vi "DrawCursorLines(SubVI).vi"(11 "CtlRef":refnum<vi>) -> (2 "Array":dbl[][](array[numeric]), 3 "reference out":refnum<vi>)   [LabVIEW 2013, in "main.lvlib"]
uses:
  main.lvlib
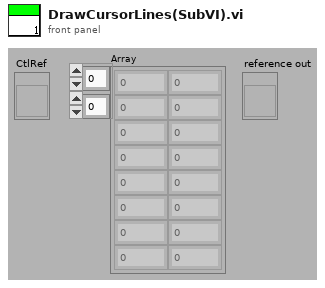
[diagram p1: front panel]
types:
  T1 = cluster{"Width":u16, "Style":enum32{"Solid", "Dash", "Dot", "DashDot", "DashDotDot"}}
  T2 = typedef "LVCursorListTypeDef.ctl" = cluster{"Name":string, "Color":u32, "Style":u8, "Point Style":u8, "Name Visible":bool, "Allow Drag":bool, "Cursor Mode":u32, "Plot":i32, "Index":i32, "Position":cluster{"X":dbl, "Y":dbl}, "X Scale":u32, "Y Scale":u32, "Watch Plots":i32[], "Watch All Plots":bool, "Plot Area":i32, "Label Offset":cluster{"X":dbl, "Y":dbl}}[]
  T3 = typedef "LVRectTypeDef.ctl" = cluster{"Left":i16, "Top":i16, "Right":i16, "Bottom":i16}
  T4 = typedef "LVPoint32TypeDef.ctl" = cluster{"Horizontal":i32, "Vertical":i32}
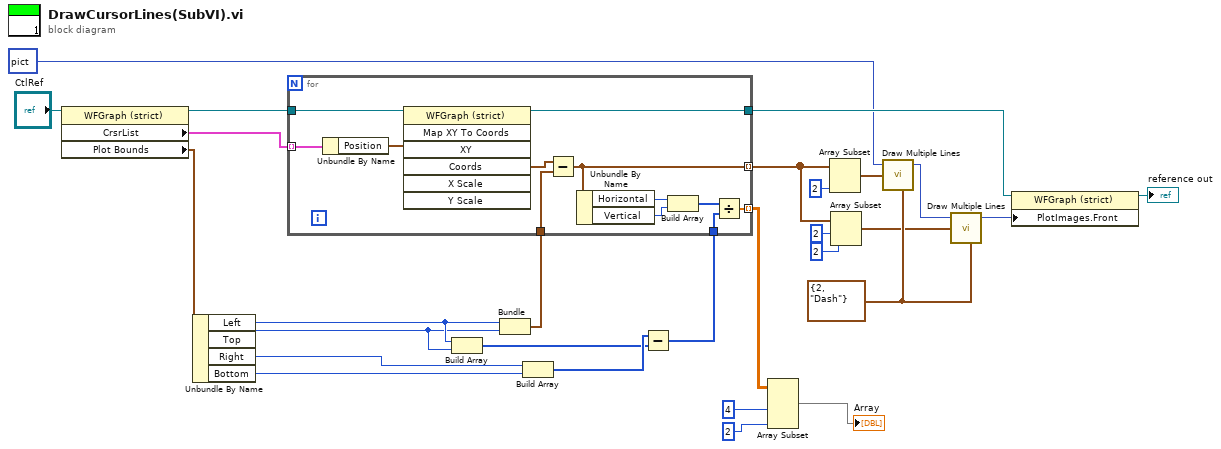
[diagram p0: block diagram]
diagram:
  w28 = T1 {"Width"=2, "Style"=enum."Dash"} ("pen")
  n1 = property class="WFGraph (strict)"(reference="CtlRef") -> (reference out=w18:refnum<vi>, "CrsrList"=w21:T2, "Plot Bounds"=w14:T3)  [unwired: 1 in, 1 out]
  n2 = Unbundle By Name(w14) -> ("Left"=w5:i16, "Top"=w4:i16, "Right"=w7:i16, "Bottom"=w8:i16)
  n3 = Build Array(w5, w4) -> (w1:i16[])
  n4 = Bundle("Left"=w5, "Top"=w4) -> (w13:cluster{"Left":i16, "Top":i16})  [unwired: 1 in]
  n5 = Build Array(w7, w8) -> (w2:i16[])
  n6 = Subtract(x=w2, y=w1) -> (x-y=w3:i16[])
  n7 = for {
    tunnel: w18 -> [w40]
    tunnel: w21 -> [w39] mode=indexing
    tunnel: w13 -> [w35]
    tunnel: [w34] -> w15 mode=indexing
    tunnel: [w37] -> w20
    tunnel: [w31] -> w6 mode=indexing
    tunnel: w3 -> [w29]
    n8 = Unbundle By Name(w39) -> ("Position"=w38:cluster{"X":dbl, "Y":dbl})
    n9 = invoke class="WFGraph (strict)" method="Map XY To Coords"(reference=w40, "XY"=w38) -> (reference out=w37:refnum<vi>, "Coords"=w36:T4)  [unwired: 5 in, 5 out]
    n10 = Subtract(x=w36, y=w35) -> (x-y=w34:T4)
    n11 = Unbundle By Name(w34) -> ("Horizontal"=w33:i32, "Vertical"=w32:i32)
    n12 = Build Array(w33, w32) -> (w30:i32[])
    n13 = Divide(x=w30, y=w29) -> (x/y=w31:dbl[])
  }
  n14 = Array Subset(array=w6, length (row)=4, length (col)=2) -> (→"Array":dbl[][])  [unwired: 2 in]
  n15 = Array Subset(array=w15, length=2) -> (w23:T4[])  [unwired: 1 in]
  n16 = Array Subset(array=w15, index=2, length=2) -> (w16:T4[])
  n17 = call <vilib>:"Draw Multiple Lines.vi"("picture"=picture data[5B] ("empty picture"), "line endpoints"=w23, "pen"=w28) -> ("new picture"=w26:picture)  [unwired: 6 in]
  n18 = call <vilib>:"Draw Multiple Lines.vi"("picture"=w26, "line endpoints"=w16, "pen"=w28) -> ("new picture"=w27:picture)  [unwired: 6 in]
  n19 = property class="WFGraph (strict)"(reference=w20, "PlotImages.Front"=w27) -> (reference out=→"reference out":refnum<vi>)  [unwired: 1 in, 1 out]
